vi "CCSA RPJ SLJC PF SubVI003.vi"(11 "Datos":T2) -> (3 "appended array":T1(array[cluster]))   [LabVIEW 2021]
doc: "Crea un arreglo de clusters, del mismo tamaño que la cantidad de muestras frontales"
panel:
  # "CUEVAS CERÓN SERGIO ALBERTO\nREYES PÉREZ JAVIER\nSALCEDO LICEA JUAN CARLOS"
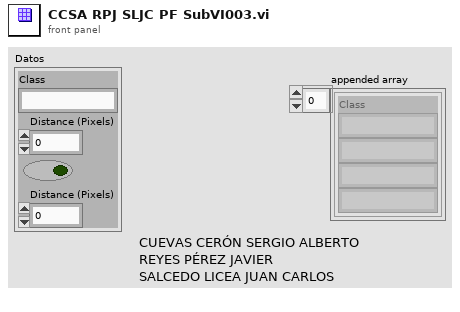
[diagram p1: front panel]
types:
  T1 = cluster{"Class":string, string, string, string}[]
  T2 = cluster{"Class":string, "Distance (Pixels)":dbl, bool, "Distance (Pixels)":dbl}
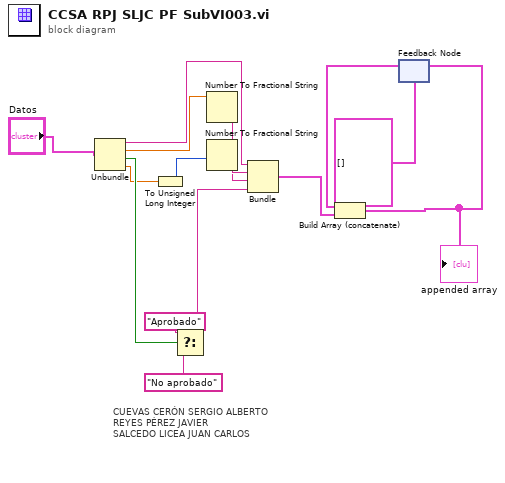
[diagram p0: block diagram]
diagram:
  # "CUEVAS CERÓN SERGIO ALBERTO\nREYES PÉREZ JAVIER\nSALCEDO LICEA JUAN CARLOS"
  n1 = Unbundle("Datos") -> ("Class"=w14:string, "Distance (Pixels)"=w10:dbl, w11:bool, "Distance (Pixels)"=w4:dbl)
  n2 = To Unsigned Long Integer(number=w4) -> (unsigned 32bit integer=w1:u32)
  n3 = Select(t="Aprobado", s=w11, f="No aprobado") -> (s? t:f=w5:string)
  n4 = Number To Fractional String(number=w10) -> (F-format string=w15:string)  [unwired: 3 in]
  n5 = Number To Fractional String(number=w1) -> (F-format string=w3:string)  [unwired: 3 in]
  n6 = Bundle("Class"=w14, w15, w3, w5) -> (w2:cluster{"Class":string, string, string, string})  [unwired: 1 in]
  n7 = feedback #1(T1 []) -> (w9:T1)
  n8 = Build Array (concatenate)(w9, w2) -> (w8:T1)
  "appended array" <- w8
  n9 = feedback-in #1(w8) -> ()
